vi "Vision Research Phantom Series PhCon PhAddIgnoredIp.vi"(2 "IpAddress":u32, 5 "Error In (no error)":errorcluster) -> (19 "Error Out":errorcluster)   [LabVIEW 2013, in "VRI.lvlib"]
doc: "PhCon.dll\n\nPhAddIgnoredIp\nHRESULT PhAddIgnoredIp(UINT IpAddress);\n\nParameters Description\nIpAddress (out) Camera IP address.\nReturn HRESULT (0 = Ok)\nComments Adds a camera IP address to the ignored list."
uses:
  VRI.lvlib
  Phantom DLLs/PhCon.Dll
panel:
  # "For instructions on the use of this VI, press Ctrl+H to display the help window and move the mouse over the icon, controls, and indicators"
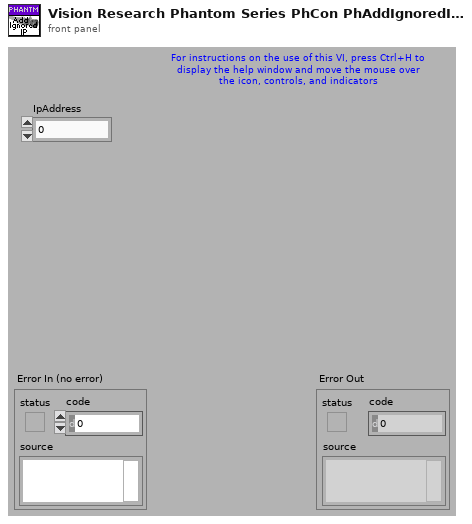
[diagram p1: front panel]
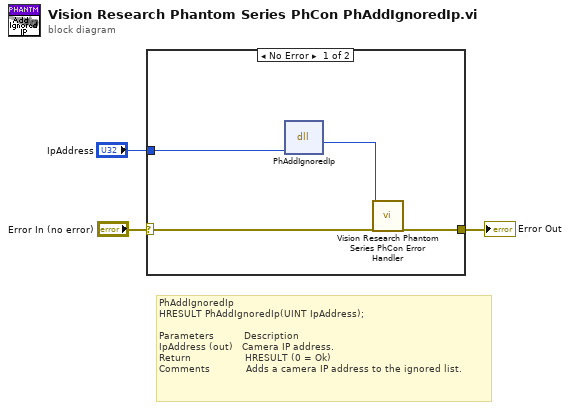
[diagram p0: block diagram]
diagram:
  # "PhAddIgnoredIp\nHRESULT PhAddIgnoredIp(UINT IpAddress);\n\nParameters          Description\nIpAddress (out)   Camera IP address.\nReturn                  HRESULT (0 = Ok)\nComments            Adds a camera IP address to the ignored list."
  n1 = case shown="No Error" "Error In (no error)" {
    selector: "Error In (no error)" -> [w7 w8]
    tunnel: [w6 w8] -> w2
    tunnel: "IpAddress" -> [w5 _]
    frame No Error {
      n2 = dll-call lib="C:/Projects/SDK/64-bit/Vision Research Phantom Series Labview Driver/Phantom DLLs/PhCon.dll" fn="PhAddIgnoredIp"("IpAddress"=w5) -> ("HRESULT"=w4:i32)  [unwired: 4 in, 2 out]
      n3 = call "Vision Research Phantom Series PhCon Error Handler.vi"("ErrNo"=w4, "Error In (no error)"=w7) -> ("Error Out"=w6:errorcluster)  [unwired: 17 out]
    }
    frame Error {
    }
  }
  "Error Out" <- w2
